vi "CANopen Heartbeat.vi"() -> ()   [LabVIEW 2016]
doc: "This example demonstrates how to read a CANopen heartbeat object."
uses:
  <vilib>/userdefined/High Color/nirio_resource_hc.ctl
  <vilib>/Platform/TimedLoop/XDataNode/timing_clust.ctl
  <vilib>/Platform/TimedLoop/XDataNode/nitl_modes.ctl
  <vilib>/Platform/TimedLoop/XDataNode/wakeup.ctl
  <vilib>/FPGAPlugInAG/cRIO-9033/niLvFpga_Open_cRIO-9033.vi
  <vilib>/rvi/interface/common/dynamic/niFpgaDynamicAddResources.vi
  <vilib>/CANopenLib/CANOPEN.llb/CANopen Interface Create.vi
  <vilib>/CANopenLib/CANOPEN.llb/CANopen SDO Create.vi
  <vilib>/CANopenLib/CANOPEN.llb/CANopen SDO Write [U16].vi
  <vilib>/CANopenLib/CANOPEN.llb/CANopen SDO Close.vi
  <vilib>/CANopenLib/CANOPEN.llb/CANopen Heartbeat Create.vi
  <vilib>/CANopenLib/CANOPEN.llb/CANopen Heartbeat Start.vi
  <vilib>/CANopenLib/CANOPEN.llb/CANopen Heartbeat State Read.vi
  <vilib>/CANopenLib/CANOPEN.llb/CANopen Heartbeat Close.vi
  <vilib>/CANopenLib/CANOPEN.llb/CANopen Interface Close.vi
  <vilib>/FPGAPlugInAG/Dynamic/niLvFpga_Close_Dynamic.vi
  <vilib>/rvi/interface/nirviOpenFPGA/nirviOpenFPGA.xnode
  FPGA Bitfiles/project_FPGATarget_MainFPGA_S9ZLErdeBuw.lvbitx
  FPGA/MainFPGA.vi
  <vilib>/Platform/TimedLoop/XDataNode/XDataNode.xnode
  <vilib>/rvi/interface/nirviCloseFPGA/nirviCloseFPGA.xnode
  <vilib>/Platform/TimedLoop/XDataNode/XDNodeRunTimeDep.lvlib
panel:
  in  "error in":errorcluster
  out "timestamp":timestamp=timestamp(3381975516.086732 s since 1904-01-01)
  out "state":u16(ring)=1 items=["unknown"=1, "boot-up"=0, "stopped"=4, "operational"=5, "pre-operational"=127, "connection lost"=128]
  in  "stop":bool
  in  "period (ms)":i64=10
  in  "consumer time (ms)":u16=1000
  in  "node-ID":u8=1 min=1 max=127 step=1
  in  "baud rate":u32(ring)=2 items=["1 Mbit/s"=0, "800 kbit/s"=1, "500 kbit/s"=2, "250 kbit/s"=3, "125 kbit/s"=4, "50 kbit/s"=6, "20 kbit/s"=7, "10 kbit/s"=8]
  in  "CANopen interface":u32(ring) items=["CANopen01", "CANopen02", "CANopen03", "CANopen04", "CANopen05", "CANopen06", "CANopen07", "CANopen08", "CANopen09", "CANopen10", "CANopen11", "CANopen12", "CANopen13", "CANopen14", "CANopen15", "CANopen16", "CANopen17", "CANopen18", "CANopen19", "CANopen20", "CANopen21", "CANopen22", "CANopen23", "CANopen24", "CANopen25", "CANopen26", "CANopen27", "CANopen28", "CANopen29", "CANopen30", "CANopen31", "CANopen32"]
  # "Overview: This example demonstrates how to read a CANopen Heartbeat object.\nRequirements: Connect CANopen module with a slave device. \nInstructions:\n1. Specify the values of CANopen interface, baud rate of the CANopen interface, node-ID of the slave device and \n    consumer time (ms) of Heartbeat object. \n2. Run this VI.\n3. Click STOP to stop the VI."
  # "Create CANopen interface and Heartbeat object"
  # "Read Heartbeat messages"
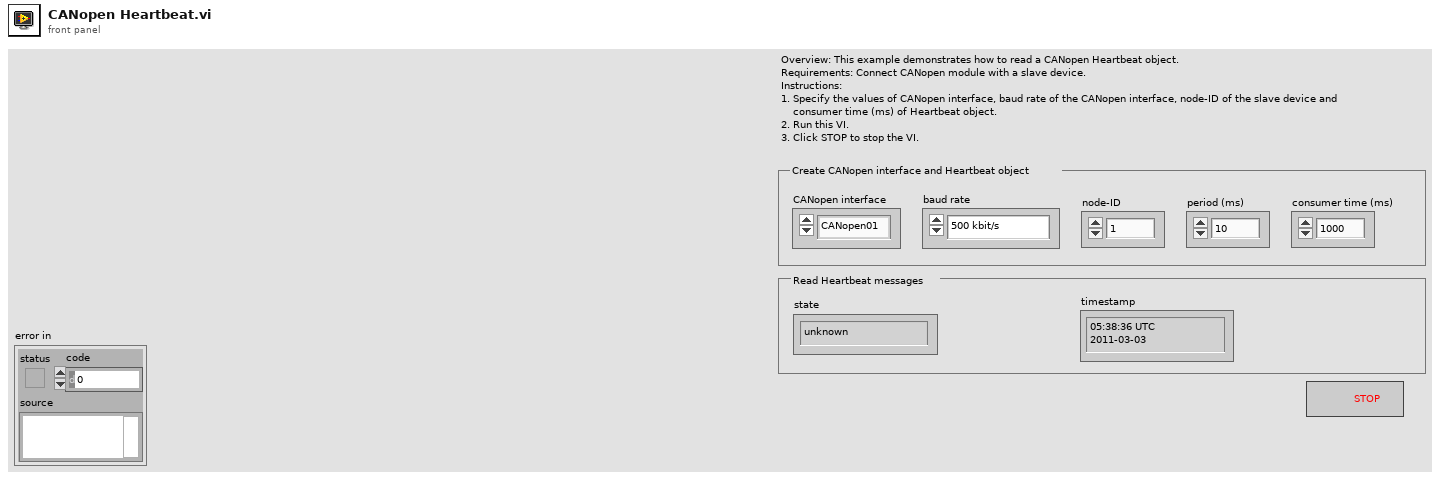
[diagram p1: front panel]
types:
  T1 = typedef "nirio_resource_hc.ctl" = tag
  T2 = typedef "XDNodeRunTimeDep.lvlib/timing_clust.ctl" = cluster{"Expected End [f-1]":u64, "Actual End [f-1]":u64, "Finished Late? [f-1]":bool, "Expected End [i-1]":u64, "Actual End [i-1]":u64, "Finished Late? [i-1]":bool, "Expected Start [i]":u64, "Actual Start [i]":u64, "Expected Start [f]":u64, "Actual Start [f]":u64, "Source Name":string, "Structure Name":string, "Period":i64, "Deadline":i64, "Offset":i64, "Start":i64, "Priority":i32, "Timeout":i32, "Mode":T3, "Wakeup Reason":T4, "Error":errorcluster, "Source Type":string, "Secondary Source Type":string, "Global End Time":u64, "Global Start Time":u64, "Frame Duration":u64, "Iteration Duration":u64, "Assigned CPU":i32, "I/O Scan Engine Mode":u32}
  T3 = typedef "XDNodeRunTimeDep.lvlib/nitl_modes.ctl" = enum32{"No Change", "Process missed periods, maintain original phase", "Discard missed periods, maintain original phase", "Process missed periods, ignore original phase", "Discard missed periods, ignore original phase"}
  T4 = typedef "XDNodeRunTimeDep.lvlib/wakeup.ctl" = enum32{"Normal", "Aborted", "Asynchronous wakeup", "Timing source error", "Timed loop error", "Timeout"}
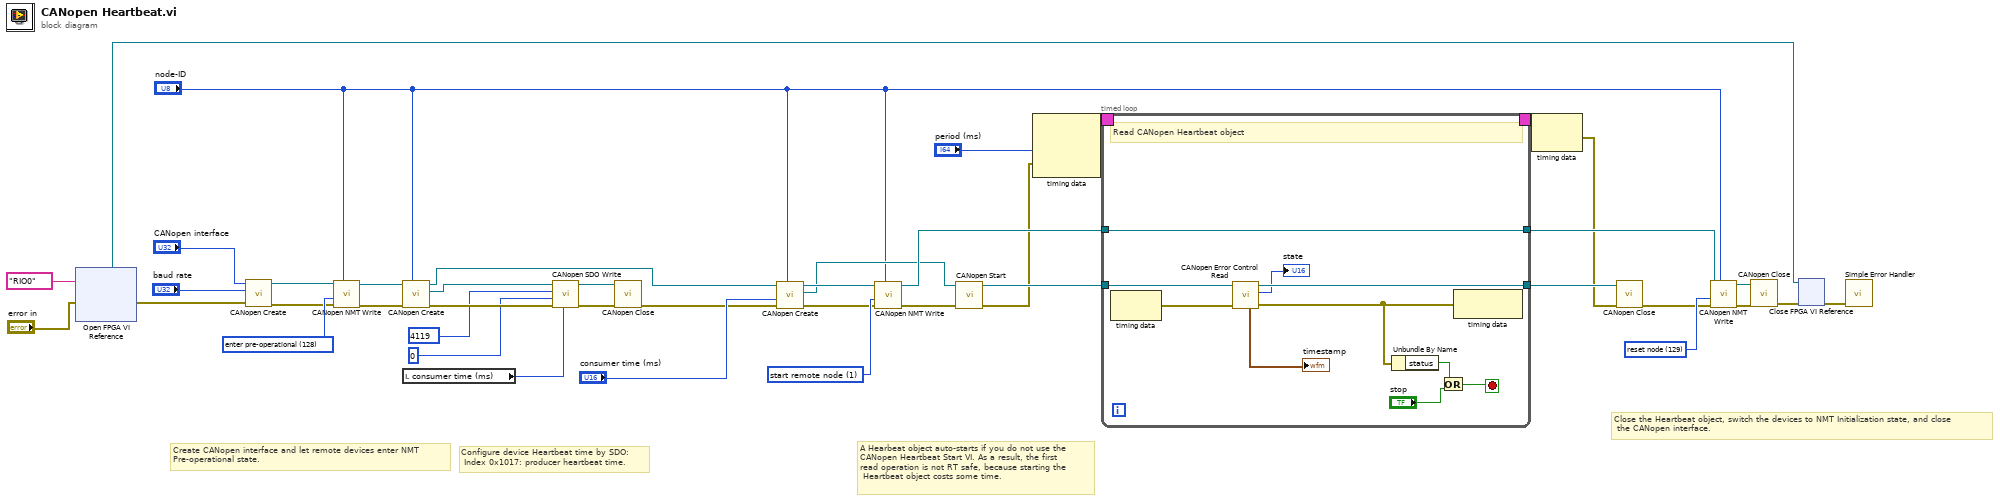
[diagram p0: block diagram]
diagram:
  w25 = u16 1 items=["start remote node"=1, "stop remote node"=2, "enter pre-operational"=128, "reset node"=129, "reset communication"=130] ("command")
  w32 = u16 129 items=["start remote node"=1, "stop remote node"=2, "enter pre-operational"=128, "reset node"=129, "reset communication"=130] ("command")
  w38 = u16 128 items=["start remote node"=1, "stop remote node"=2, "enter pre-operational"=128, "reset node"=129, "reset communication"=130] ("command")
  # "A Hearbeat object auto-starts if you do not use the \nCANopen Heartbeat Start VI. As a result, the first \nread operation is not RT safe, because starting the\n Heartbeat object costs some time."
  # "Close the Heartbeat object, switch the devices to NMT Initialization state, and close\n the CANopen interface."
  # "Create CANopen interface and let remote devices enter NMT\nPre-operational state."
  # "Configure device Heartbeat time by SDO:\n Index 0x1017: producer heartbeat time."
  n1 = xnode ("Open FPGA VI Reference")("error in"="error in", "resource name"=T1 "RIO0") -> ("FPGA VI Reference Out"=w1:refnum<k20>, "error out"=w4:errorcluster)
  n2 = call-poly <vilib>:"CANopen Create.vi"("error in (no error)"=w4, "baud rate"="baud rate", "interface name"="CANopen interface") -> ("error out"=w37:errorcluster, "interface object out"=w36:refnum<k20>)  [unwired: 7 in]
  n3 = call <vilib>:"CANopen NMT Write.vi"("node-ID (0)"="node-ID", "error in (no error)"=w37, "command"=w38, "interface object in"=w36) -> ("error out"=w20:errorcluster, "interface object out"=w23:refnum<k20>)  [unwired: 6 in]
  n4 = call-poly <vilib>:"CANopen Create.vi"("node-ID"="node-ID", "error in (no error)"=w20, "interface object in"=w23) -> ("error out"=w19:errorcluster, "SDO object out"=w21:refnum<k20>, "interface object out"=w22:refnum<k20>)  [unwired: 6 in]
  n5 = local read "consumer time (ms)"() -> (w13:u16)
  n6 = call-poly <vilib>:"CANopen SDO Write.vi"("U16 data"=w13, "error in (no error)"=w19, "object sub-index (0)"=u8 0, "object index"=u16 4119, "SDO object in"=w21) -> ("error out"=w18:errorcluster, "SDO object out"=w15:refnum<k20>)  [unwired: 4 in, 1 out]
  n7 = call-poly <vilib>:"CANopen Close.vi"("error in (no error)"=w18, "SDO object in"=w15) -> ("error out"=w17:errorcluster)  [unwired: 9 in]
  n8 = call-poly <vilib>:"CANopen Create.vi"("node-ID"="node-ID", "error in (no error)"=w17, "consumer time [ms]"="consumer time (ms)", "interface object in"=w22) -> ("error out"=w12:errorcluster, "heartbeat object out"=w11:refnum<k20>, "interface object out"=w27:refnum<k20>)  [unwired: 5 in]
  n9 = call <vilib>:"CANopen NMT Write.vi"("node-ID (0)"="node-ID", "error in (no error)"=w12, "command"=w25, "interface object in"=w27) -> ("error out"=w24:errorcluster, "interface object out"=w26:refnum<k20>)  [unwired: 6 in]
  n10 = call-poly <vilib>:"CANopen Start.vi"("error in (no error)"=w24, "heartbeat object in"=w11) -> ("error out"=w9:errorcluster, "heartbeat object out"=w33:refnum<k20>)  [unwired: 8 in]
  n11 = node-c288("period (ms)", w9) -> (w42:T2)  [unwired: 1 in]
  n12 = timed-loop {
    tunnel: w33 -> [w51]
    tunnel: [w50] -> w35
    tunnel: w26 -> [w48]
    tunnel: [w48] -> w28
    timing: w42 -> [_]
    timing-out: [_] -> w41
    stop <- w45 stop-if-true
    # "Read CANopen Heartbeat object"
    n13 = node-c288() -> (w47:errorcluster)  [unwired: 1 in]
    n14 = call-poly <vilib>:"CANopen Error Control Read.vi"("error in (no error)"=w47, "heartbeat object in"=w51) -> ("error out"=w46:errorcluster, "state"=→"state":u16, "heartbeat object out"=w50:refnum<k20>, "timestamp"=→"timestamp":timestamp)  [unwired: 6 in]
    n15 = Unbundle By Name(w46) -> ("status"=w44:bool)
    n16 = Or(x=w44, y="stop") -> (x .or. y?=w45:bool)
    n17 = node-c288(w46) -> ()  [unwired: 1 out]
  }
  n18 = node-c288(w41) -> (w8:errorcluster)
  n19 = call-poly <vilib>:"CANopen Close.vi"("error in (no error)"=w8, "heartbeat object in"=w35) -> ("error out"=w29:errorcluster)  [unwired: 9 in]
  n20 = call <vilib>:"CANopen NMT Write.vi"("node-ID (0)"="node-ID", "error in (no error)"=w29, "command"=w32, "interface object in"=w28) -> ("error out"=w30:errorcluster, "interface object out"=w31:refnum<k20>)  [unwired: 6 in]
  n21 = call-poly <vilib>:"CANopen Close.vi"("error in (no error)"=w30, "interface object in"=w31) -> ("error out"=w3:errorcluster)  [unwired: 9 in]
  n22 = xnode "Close FPGA VI Reference"("FPGA VI Reference In"=w1, "error in"=w3) -> ("error out"=w2:errorcluster)
  n23 = call <vilib>:"Simple Error Handler.vi"("error in (no error)"=w2) -> ()  [unwired: 4 in, 5 out]
